vi "DEV Read User Data.vi"(7 "DataLen":i32, 9 "pReadData":u8, 10 "OffsetAddr":i32, 11 "DevHandle":i32) -> (1 "pReadData out":u8, 3 "function return":bool)   [LabVIEW 2010, in "usb_device.lvlib"]
doc: "bool WINAPI DEV_ReadUserData(int DevHandle,int OffsetAddr,unsigned char *pReadData,int DataLen);"
uses:
  usb_device.lvlib
  USB2XXX.dll
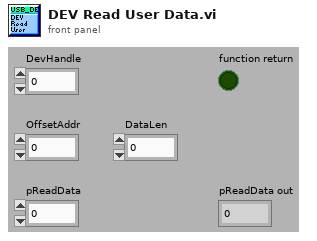
[diagram p1: front panel]
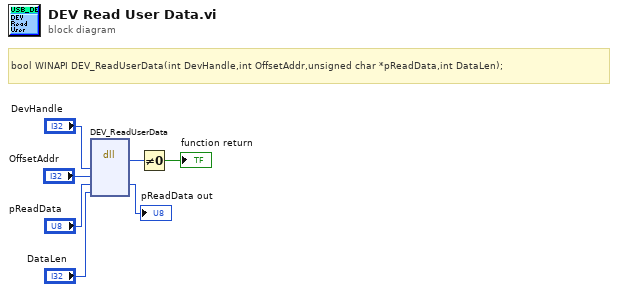
[diagram p0: block diagram]
diagram:
  # "bool WINAPI DEV_ReadUserData(int DevHandle,int OffsetAddr,unsigned char *pReadData,int DataLen);"
  n1 = dll-call lib="G:/OtherWork/USB2XXX_Example/trunk/Labview/PublicFiles/usb_device/USB2XXX.*" fn="DEV_ReadUserData"("DevHandle"="DevHandle", "OffsetAddr"="OffsetAddr", "pReadData"="pReadData", "DataLen"="DataLen") -> (w6:u8, "pReadData"=→"pReadData out":u8)  [unwired: 6 in, 2 out]
  n2 = Not Equal To 0?(x=w6) -> (x != 0?=→"function return":bool)
